vi "Count Up U32.vi"(0 "increment":bool=TRUE, 1 "reset":bool) -> (4 "count out":u32)   [LabVIEW 2013, in "Engine Simulation Toolkit.lvlib"]
uses:
  Engine Simulation Toolkit.lvlib
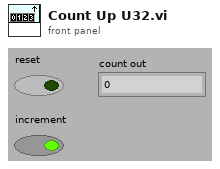
[diagram p1: front panel]
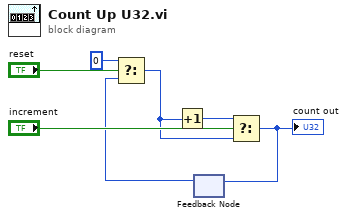
[diagram p0: block diagram]
diagram:
  n1 = feedback #1() -> (w3:u32)  [unwired: 1 in]
  n2 = Select(t=u32 0 ("count in"), s="reset", f=w3) -> (s? t:f=w2:u32)
  n3 = Increment(x=w2) -> (x+1=w4:u32)
  n4 = Select(t=w4, s="increment", f=w2) -> (s? t:f=w1:u32)
  "count out" <- w1
  n5 = feedback-in #1(w1) -> ()
